vi "processCommandPublish.vi"(8 "error in (no error)":errorcluster, 11 "MiddlewareSVThisComponent in":refnum<class "MiddlewareSVThisComponent.lvclass">) -> (0 "error out":errorcluster, 3 "MiddlewareSVThisComponent out":refnum<class "MiddlewareSVThisComponent.lvclass">)   [LabVIEW 2016, in "MiddlewareSVThisComponent.lvclass"]
uses:
  MiddlewareSVThisComponent.lvclass
  ComponentTemplateCore/ComponentModel/ComponentModel/MiddlewareSV/MiddlewareSV.lvclass
  <vilib>/Utility/error.llb/DialogType.ctl
  ComponentTemplateCore/ComponentModel/ComponentModel/Middleware/Middleware.lvclass
  ComponentTemplateCore/ComponentModel/ComponentModel/CommandEvent/CommandEvent.lvclass
  ComponentTemplateCore/ComponentModel/ComponentModel/MiddlewareProcessEvent/MiddlewareProcessEvent.lvclass
  home/andres/ct_cmpuserevents/ComponentTemplateCore/ComponentModel/ComponentModel/MiddlewareSV/MiddlewareSV.lvclass
  home/andres/ct_cmpuserevents/ComponentTemplateCore/ComponentModel/ComponentModel/Middleware/Middleware.lvclass
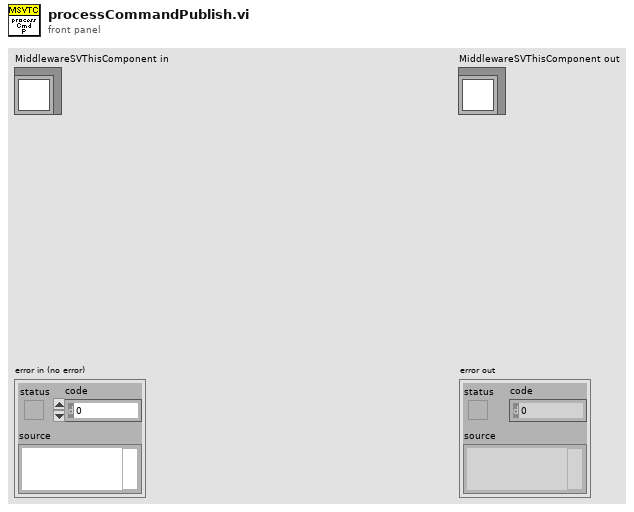
[diagram p1: front panel]
types:
  T1 = typedef "EXATypedefs.lvlib/CommandEvents.ctl" = cluster{"command":refnum<user-event>}
  T2 = typedef "MiddlewareProcessEvents.ctl" = cluster{"disconnect":refnum<user-event>, "error":refnum<user-event>}
  T3 = typedef "DialogType.ctl" = u16
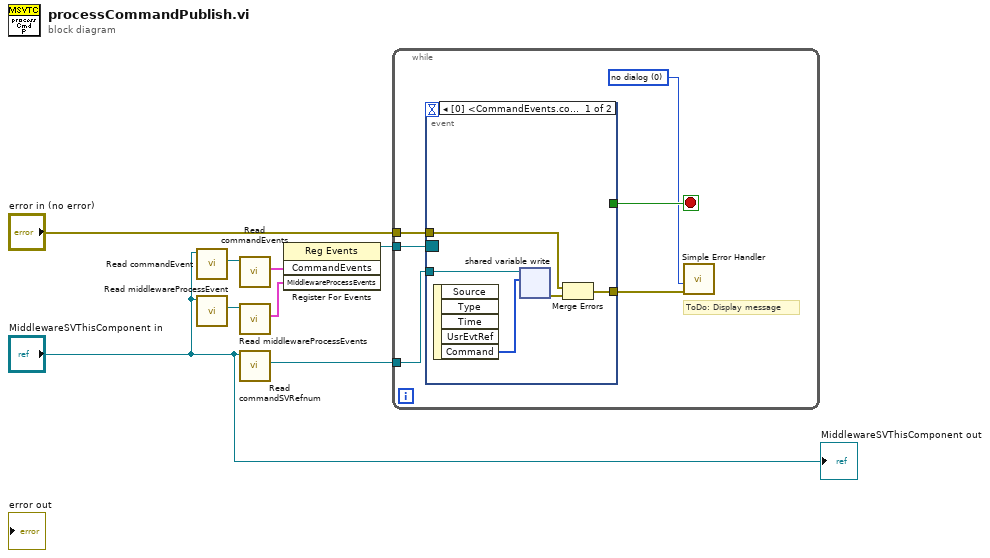
[diagram p0: block diagram]
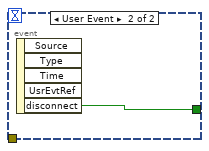
[diagram p2: hidden frame]
diagram:
  n1 = call "Read commandEvent.vi"("Middleware in"="MiddlewareSVThisComponent in") -> ("commandEvent"=w5:refnum<class "CommandEvent.lvclass">)  [unwired: 9 in, 1 out]
  n2 = call "Read middlewareProcessEvent.vi"("Middleware in"="MiddlewareSVThisComponent in") -> ("middlewareProcessEvent"=w2:refnum<class "MiddlewareProcessEvent.lvclass">)  [unwired: 9 in, 1 out]
  n3 = call "Read commandEvents.vi"("CommandEvent in"=w5) -> ("CommandEvents"=w4:T1)  [unwired: 9 in, 1 out]
  n4 = call "Read middlewareProcessEvents.vi"("MiddlewareProcessEvent in"=w2) -> ("MiddlewareProcessEvents"=w1:T2)  [unwired: 9 in, 1 out]
  n5 = call "Read commandSVRefnum.vi"("MiddlewareSV in"="MiddlewareSVThisComponent in") -> ("commandSVRefnum"=w7:refnum<k21>)  [unwired: 9 in, 1 out]
  n6 = register-events(w4, w1) -> (reference out=w8:refnum<event-registration>)  [unwired: 2 in, 1 out]
  n7 = while {
    tunnel: w8 -> [w14]
    tunnel: w7 -> [w12]
    tunnel: "error in (no error)" -> [w10]
    stop <- w13 stop-if-true
    w11 = T3 0 items=["no dialog", "OK message", "continue or stop message", "OK message + warnings", "continue/stop + warnings"] ("type of dialog (OK msg:1)")
    # "ToDo: Display message"
    n8 = event shown="[0] <CommandEvents.command>: User Event" {
      selector: w14 -> [_ _]
      dyn-events: _ -> [_ _]
      timeout: _ -> [_ _]
      tunnel: [_ w20] -> w13
      tunnel: w12 -> [w18 _]
      tunnel: w10 -> [w17 _]
      tunnel: [w15 _] -> w9
      event User Event {
        n9 = event-data() -> ("Command"=w19:u8[])  [unwired: 1 in, 4 out]
        n10 = shared-variable-write(w18, w19) -> (w16:errorcluster)  [unwired: 1 in, 1 out]
        n11 = Merge Errors(w17, w16) -> (w15:errorcluster)
      }
      event User Event {
        n12 = event-data() -> ("disconnect"=w20:bool)  [unwired: 1 in, 4 out]
      }
    }
    n13 = call <vilib>:"Simple Error Handler.vi"("type of dialog (OK msg:1)"=w11, "error in (no error)"=w9) -> ()  [unwired: 3 in, 5 out]
  }
  "MiddlewareSVThisComponent out" <- "MiddlewareSVThisComponent in"
